vi "Initialize.vi"(8 "error in (no error)":errorcluster, 9 "reset":bool=TRUE, 10 "ID query":bool=TRUE, 11 "VISA resource name":refnum<visa-resource-name>="GPIB::16") -> (0 "error out":errorcluster, 3 "VISA resource name out":refnum<visa-resource-name>)   [LabVIEW 2018, in "Agilent 87XX Series.lvlib"]
doc: "This VI loads the addressing information about the instrument into the Open VXI Instrument VI and returns the instrument ID. You can reset the instrument by setting the front panel reset control. You must run this VI before using any of the instrument driver VIs for this instrument.\n\nFor the HP8753, make the instrument descriptor \"GPIB::16\" or whatever the primary address of your instrument is."
uses:
  Agilent 87XX Series.lvlib
panel:
  # "© 2005 National Instruments.  ALL RIGHTS RESERVED."
  # "yes\nno"
  # "yes\nno"
  # "Performing the instrument\nquery is recommended with\nall HP8753s. To understand\nwhy, read the text on this\nVI's diagram."
  # "After running the initialize VI, you must do one of two things. First, \nyou can copy data out of the \"VISA session\" indicator and paste \nit into the \"VISA session\" of the VI you want to run. Alternately when\nyou are using several VIs together, you can wire the \"VISA session\" \nof one VI to the \"VISA session\" of another VI as in the \"EXAMPLE\" \nVI. Without, the \"VISA session\", a VI will not run. Running a VI without\n the \"VISA session\" will generate a error coded -1232."
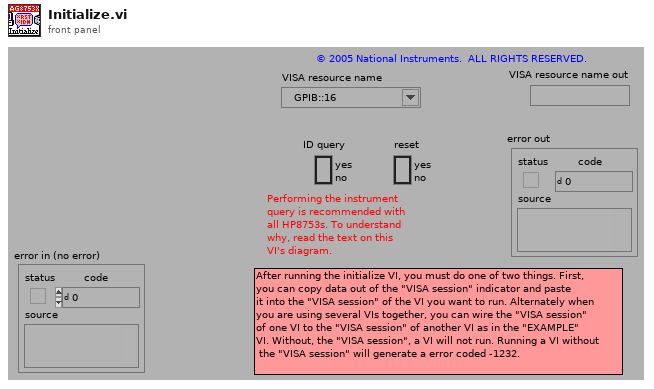
[diagram p1: front panel]
types:
  T1 = cluster{"status":bool, "code":i32, "VI name":string}
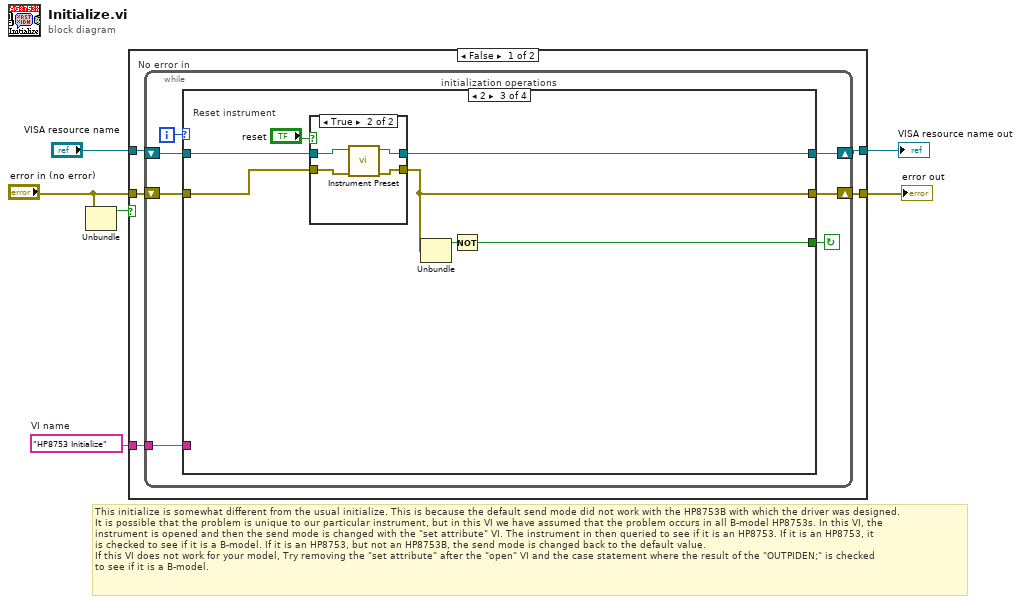
[diagram p0: block diagram]
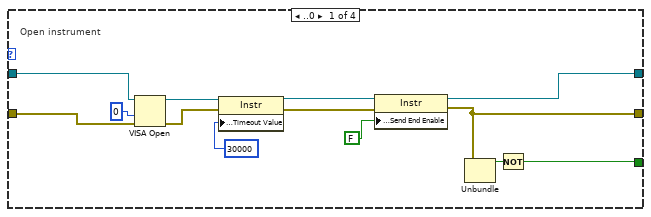
[diagram p2: hidden frame]
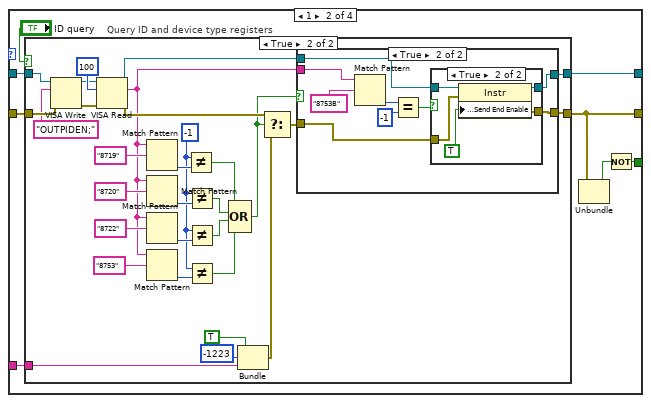
[diagram p3: hidden frame]
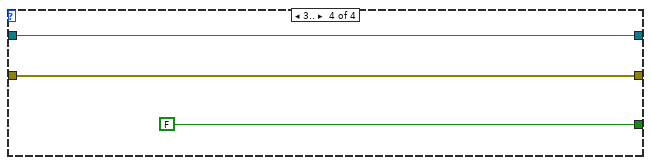
[diagram p8: hidden frame]
diagram:
  w6 = "HP8753 Initialize"  # VI name
  # "This initialize is somewhat different from the usual initialize. This is because the default send mode did not work with the HP8753B with which the driver was designed.\nIt is possible that the problem is unique to our particular instrument, but in this VI we have assumed that the problem occurs in all B-model HP8753s. In this VI, the \ninstrument is opened and then the send mode is changed with the \"set attribute\" VI. The instrument in then queried to see if it is an HP8753. If it is an HP8753, it\nis checked to see if it is a B-model. If it is an HP8753, but not an HP8753B, the send mode is changed back to the default value.\nIf this VI does not work for your model, Try removing the \"set attribute\" after the \"open\" VI and the case statement where the result of the \"OUTPIDEN;\" is checked\nto see if it is a B-model."
  n1 = Unbundle("error in (no error)") -> ("status"=w5:bool)  [unwired: 2 out]
  n2 = case shown="False" w5 {
    tunnel: "error in (no error)" -> [w11 w107]
    tunnel: w6 -> [w10 _]
    tunnel: [w9 w107] -> w4
    tunnel: [w8 w106] -> w2
    tunnel: "VISA resource name" -> [w7 w106]
    frame False {
      # "No error in"
      n3 = while {
        tunnel: w10 -> [w13]
        shift-left: w7 -> [w14]
        shift-right: [w15] -> w8
        shift-left: w11 -> [w18]
        shift-right: [w17] -> w9
        i -> [w16]
        stop <- w12 continue-if-true
        n4 = case "initialization operations" shown="2" w16 {
          tunnel: w18 -> [w21 w39 w96 w104]
          tunnel: [w28 w34 w92 w104] -> w17
          tunnel: [w27 w37 w93 w103] -> w15
          tunnel: w14 -> [w20 w38 w94 w103]
          tunnel: w13 -> [_ w35 _ _]
          tunnel: [w31 w32 w90 FALSE] -> w12
          frame ..0 {
            # "Open instrument"
            n5 = VISA Open(access mode=u32 0, error in (no error)=w21, VISA resource name=w20) -> (VISA resource name=w23:refnum<visa-resource-name>, error out=w22:errorcluster)  [unwired: 2 in]
            n6 = property class="Instr"(reference=w23, error in=w22, "General Settings:Timeout Value"=u32 30000 ("Tmo Value")) -> (reference out=w24:refnum<visa-resource-name>, error out=w25:errorcluster)
            n7 = property class="Instr"(reference=w24, error in=w25, "Message Based Settings:Send End Enable"=FALSE) -> (reference out=w27:refnum<visa-resource-name>, error out=w28:errorcluster)
            n8 = Unbundle(w28) -> ("status"=w29:bool)  [unwired: 2 out]
            n9 = Not(x=w29) -> (.not. x?=w31:bool)
          }
          frame 1 {
            # "Query ID and device type registers"
            n10 = case shown="True" "ID query" {
              tunnel: [w40 w60] -> w34
              tunnel: w39 -> [w40 w67]
              tunnel: [w41 w58] -> w37
              tunnel: w38 -> [w41 w57]
              tunnel: w35 -> [_ w68]
              frame False {
              }
              frame True {
                w43 = -1 ("x")
                n11 = VISA Write(VISA resource name=w57, write buffer="OUTPIDEN;", error in (no error)=w67) -> (VISA resource name out=w61:refnum<visa-resource-name>, error out=w65:errorcluster)  [unwired: 1 out]
                n12 = VISA Read(VISA resource name=w61, byte count=u32 100, error in (no error)=w65) -> (VISA resource name out=w63:refnum<visa-resource-name>, read buffer=w44:string, error out=w64:errorcluster)  [unwired: 1 out]
                n13 = Match Pattern(string=w44, regular expression="8719") -> (offset past match=w52:i32)  [unwired: 1 in, 3 out]
                n14 = Match Pattern(string=w44, regular expression="8720") -> (offset past match=w51:i32)  [unwired: 1 in, 3 out]
                n15 = Match Pattern(string=w44, regular expression="8722") -> (offset past match=w50:i32)  [unwired: 1 in, 3 out]
                n16 = Match Pattern(string=w44, regular expression="8753") -> (offset past match=w49:i32)  [unwired: 1 in, 3 out]
                n17 = Not Equal?(x=w43, y=w52) -> (x != y?=w48:bool)
                n18 = Not Equal?(x=w43, y=w51) -> (x != y?=w45:bool)
                n19 = Not Equal?(x=w43, y=w50) -> (x != y?=w46:bool)
                n20 = Not Equal?(x=w43, y=w49) -> (x != y?=w47:bool)
                n21 = Compound Arithmetic op=OR(w48, w45, w46, w47) -> (w42:bool)
                n22 = Bundle(TRUE, -1223, "VI name"=w68) -> (w69:cluster{bool, i32, "VI name":string})  [unwired: 1 in]
                n23 = Select(t=w64, s=w42, f=w69) -> (s? t:f=w59:T1)
                n24 = case shown="True" w42 {
                  tunnel: w63 -> [w72 w76]
                  tunnel: [w73 w77] -> w60
                  tunnel: w59 -> [w73 w78]
                  tunnel: w44 -> [_ w75]
                  tunnel: [w72 w74] -> w58
                  frame False {
                  }
                  frame True {
                    n25 = Match Pattern(string=w75, regular expression="8753B") -> (offset past match=w81:i32)  [unwired: 1 in, 3 out]
                    n26 = Equal?(x=w81, y=-1) -> (x = y?=w79:bool)
                    n27 = case shown="True" w79 {
                      tunnel: w78 -> [w84 w89]
                      tunnel: [w84 w88] -> w77
                      tunnel: w76 -> [w83 w87]
                      tunnel: [w83 w85] -> w74
                      frame False {
                      }
                      frame True {
                        n28 = property class="Instr"(reference=w87, error in=w89, "Message Based Settings:Send End Enable"=TRUE) -> (reference out=w85:refnum<visa-resource-name>, error out=w88:errorcluster)
                      }
                    }
                  }
                }
              }
            }
            n29 = Unbundle(w34) -> ("status"=w33:bool)  [unwired: 2 out]
            n30 = Not(x=w33) -> (.not. x?=w32:bool)
          }
          frame 2 {
            # "Reset instrument"
            n31 = case shown="True" "reset" {
              tunnel: w96 -> [w98 w102]
              tunnel: [w98 w101] -> w92
              tunnel: w94 -> [w97 w100]
              tunnel: [w97 w99] -> w93
              frame False {
              }
              frame True {
                n32 = call "Instrument Preset.vi"("error in (no error)"=w102, "VISA resource name"=w100) -> ("error out"=w101:errorcluster, "VISA resource name out"=w99:refnum<visa-resource-name>)  [unwired: 8 in]
              }
            }
            n33 = Unbundle(w92) -> ("status"=w91:bool)  [unwired: 2 out]
            n34 = Not(x=w91) -> (.not. x?=w90:bool)
          }
          frame 3.. {
          }
        }
      }
    }
    frame True {
      # "Error"
    }
  }
  "VISA resource name out" <- w2
  "error out" <- w4
